vi "DuplicateArray.vi"(9 "Array":dbl[](array[numeric]), 10 "Number of frames":i32) -> (2 "Duplicated Array":dbl[](array[numeric]))   [LabVIEW 2015]
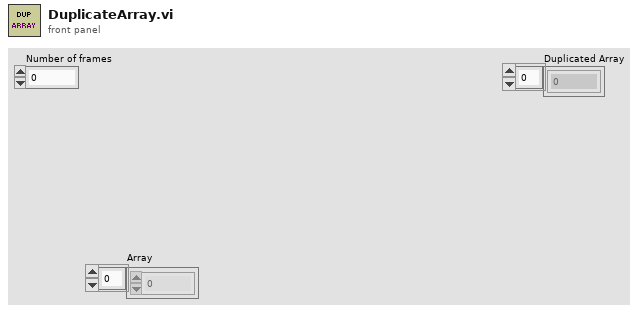
[diagram p1: front panel]
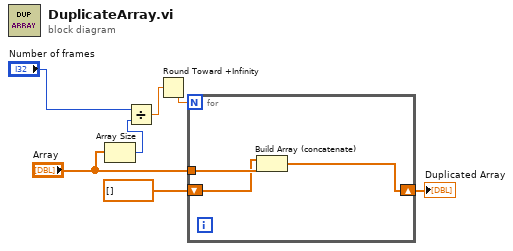
[diagram p0: block diagram]
diagram:
  n1 = Array Size(array="Array") -> (size(s)=w4:i32)
  n2 = Divide(x="Number of frames", y=w4) -> (x/y=w2:dbl)
  n3 = Round Toward +Infinity(x=w2) -> (ceil(x): smallest int >= x=w1:dbl)
  n4 = for {
    N: w1 -> [_]
    tunnel: "Array" -> [w10]
    shift-right: [w8] -> w6
    shift-left: dbl[] [] ("Array") -> [w9]
    n5 = Build Array (concatenate)(w9, w10) -> (w8:dbl[])
  }
  "Duplicated Array" <- w6
